vi "C37 Get Phasor Configuration.vi"(8 "error in (no error)":errorcluster, 9 "Phasor Index":i32, 10 "PMU Index":i32, 11 "Pseudo PDC ID":i32) -> (0 "error out":errorcluster, 2 "Channel Name":string, 3 "Phasor Configuration":T1)   [LabVIEW 2013, in "C37118-DLL.lvlib"]
uses:
  C37118-DLL.lvlib
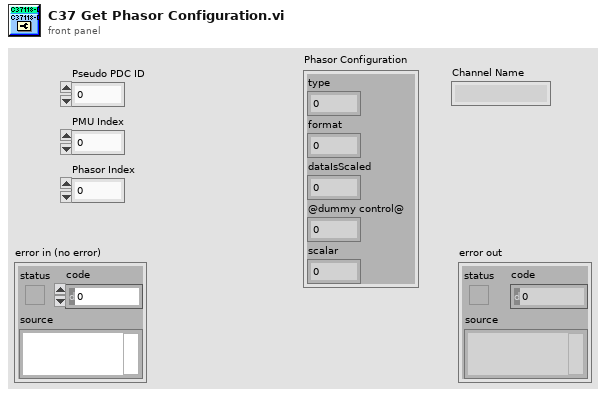
[diagram p1: front panel]
types:
  T1 = cluster{"type":u8, "format":u8, "dataIsScaled":u8, "@dummy control@":i8, "scalar":sgl}
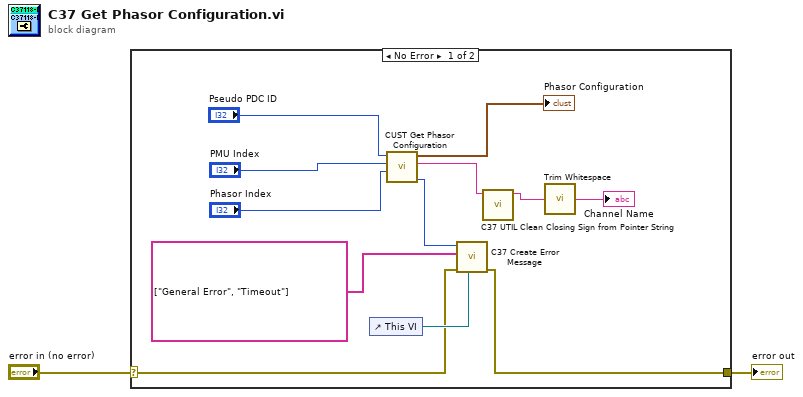
[diagram p0: block diagram]
diagram:
  n1 = case shown="No Error" "error in (no error)" {
    selector: "error in (no error)" -> [w13 w15]
    tunnel: [w12 w15] -> w2
    frame No Error {
      n2 = control-ref of="This VI"() -> (w14:refnum<vi>)
      n3 = call "CUST Get Phasor Configuration.vi"("phasorIndex"="Phasor Index", "pmuIndex"="PMU Index", "pseudoPdcId"="Pseudo PDC ID") -> ("function return"=w4:i32, "name out"=w3:string, "phasorCfg out"=→"Phasor Configuration":T1)  [unwired: 6 in]
      n4 = call "C37 Create Error Message.vi"("VI Reference"=w14, "error in (no error)"=w13, "Error Messages"=string[] ["General Error", "Timeout"], "function return"=w4) -> ("error out"=w12:errorcluster)  [unwired: 7 in]
      n5 = call "C37 UTIL Clean Closing Sign from Pointer String.vi"("String In"=w3) -> ("String Out"=w9:string)  [unwired: 10 in]
      n6 = call <vilib>:"Trim Whitespace.vi"("string"=w9) -> ("trimmed string"=→"Channel Name":string)  [unwired: 1 in]
    }
    frame Error {
    }
  }
  "error out" <- w2
